vi "Bundle EQ and Z Graphs.vi"(4 "Frequency":dbl, 6 "1D Frequency In":dbl[](array[numeric]), 8 "1D Impedance In":dbl[](array[numeric]), 9 "2D Impedandce In":dbl[][](array[numeric]), 10 "2D Gain In":dbl[][](array[numeric]), 11 "1D Gain In":dbl[](array[numeric])) -> (0 "1D Frequency Out":dbl[](array[numeric]), 1 "2D Impedandce Out":dbl[][](array[numeric]), 2 "2D Gain Out":dbl[][](array[numeric]), 3 "Z Graph":cluster{dbl[], dbl[]}[](array[cluster]), 7 "EQ Graph":cluster{dbl[], dbl[]}[](array[cluster]))   [LabVIEW 2021]
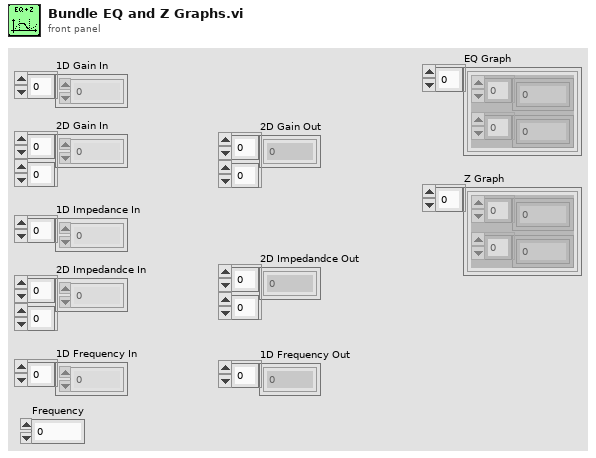
[diagram p1: front panel]
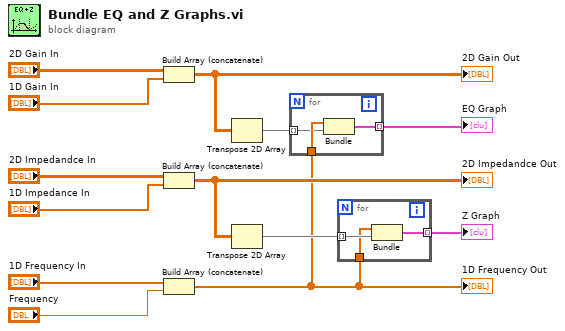
[diagram p0: block diagram]
diagram:
  n1 = Build Array (concatenate)("2D Gain In", "1D Gain In") -> (w5:dbl[][])
  "2D Gain Out" <- w5
  n2 = Build Array (concatenate)("2D Impedandce In", "1D Impedance In") -> (w4:dbl[][])
  "2D Impedandce Out" <- w4
  n3 = Build Array (concatenate)("1D Frequency In", "Frequency") -> (w3:dbl[])
  "1D Frequency Out" <- w3
  n4 = Transpose 2D Array(2D array=w5) -> (transposed array=w7:dbl[][])
  n5 = Transpose 2D Array(2D array=w4) -> (transposed array=w6:dbl[][])
  n6 = for {
    tunnel: w3 -> [w16]
    tunnel: w7 -> [w15] mode=indexing
    tunnel: [w14] -> w2 mode=indexing
    n7 = Bundle(w16, w15) -> (w14:cluster{dbl[], dbl[]})  [unwired: 1 in]
  }
  "EQ Graph" <- w2
  n8 = for {
    tunnel: w6 -> [w19] mode=indexing
    tunnel: w3 -> [w18]
    tunnel: [w17] -> w1 mode=indexing
    n9 = Bundle(w18, w19) -> (w17:cluster{dbl[], dbl[]})  [unwired: 1 in]
  }
  "Z Graph" <- w1
